vi "testtime.vi"() -> ()   [LabVIEW 2022 SP3]
panel:
  out "error out 8":errorcluster
  out "error out 7":errorcluster
  out "error out 6":errorcluster
  out "error out 5":errorcluster
  out "error out 4":errorcluster
  out "1 28":dbl format="%04d"
  out "1 27":dbl format="%04d"
  out "1 26":dbl format="%04d"
  out "1 25":dbl format="%04d"
  out "1 24":dbl format="%04d"
  out "1 23":dbl format="%04d"
  out "1 22":dbl format="%04d"
  out "error out 3":errorcluster
  out "1 21":dbl format="%04d"
  out "1 20":dbl format="%04d"
  out "1 19":dbl format="%04d"
  out "1 18":dbl format="%04d"
  out "1 17":dbl format="%04d"
  out "1 16":dbl format="%04d"
  out "1 15":dbl format="%04d"
  out "1 14":dbl format="%04d"
  out "1 13":dbl format="%04d"
  out "1 12":dbl format="%04d"
  out "1 11":dbl format="%04d"
  out "1 10":dbl format="%04d"
  out "1 9":dbl format="%04d"
  out "1 8":dbl format="%04d"
  out "error out 2":errorcluster
  in  "8":bool
  out "1 7":dbl format="%04d"
  out "1 6":dbl format="%04d"
  out "1 5":dbl format="%04d"
  out "1 4":dbl format="%04d"
  out "1 3":dbl format="%04d"
  out "1 2":dbl format="%04d"
  out "1":dbl format="%04d"
  out "error out":errorcluster
  # "A"
  # "B"
  # "C"
  # "D"
  # "11."
  # "Time"
  # "Setting"
  # "12."
  # "13."
  # "14."
  # "15."
  # "16."
  # "21."
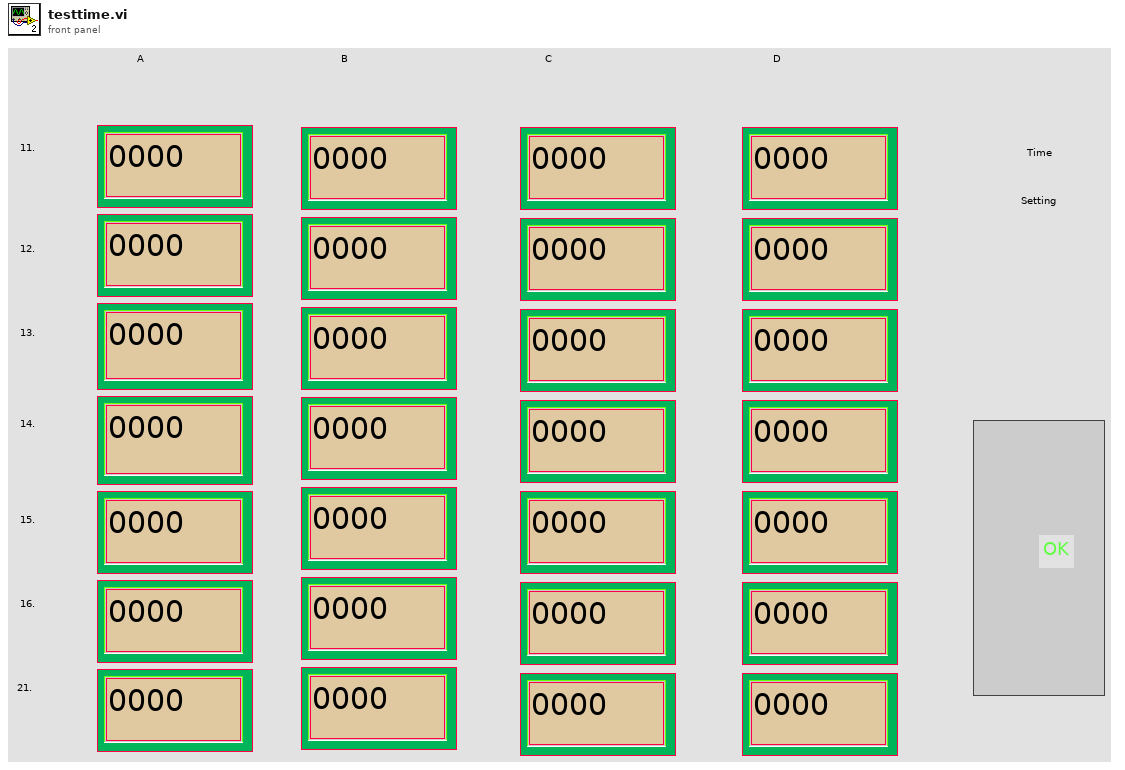
[diagram p1: front panel]
types:
  T1 = enum16{"open", "replace", "create", "open or create", "replace or create", "replace or create with confirmation"}
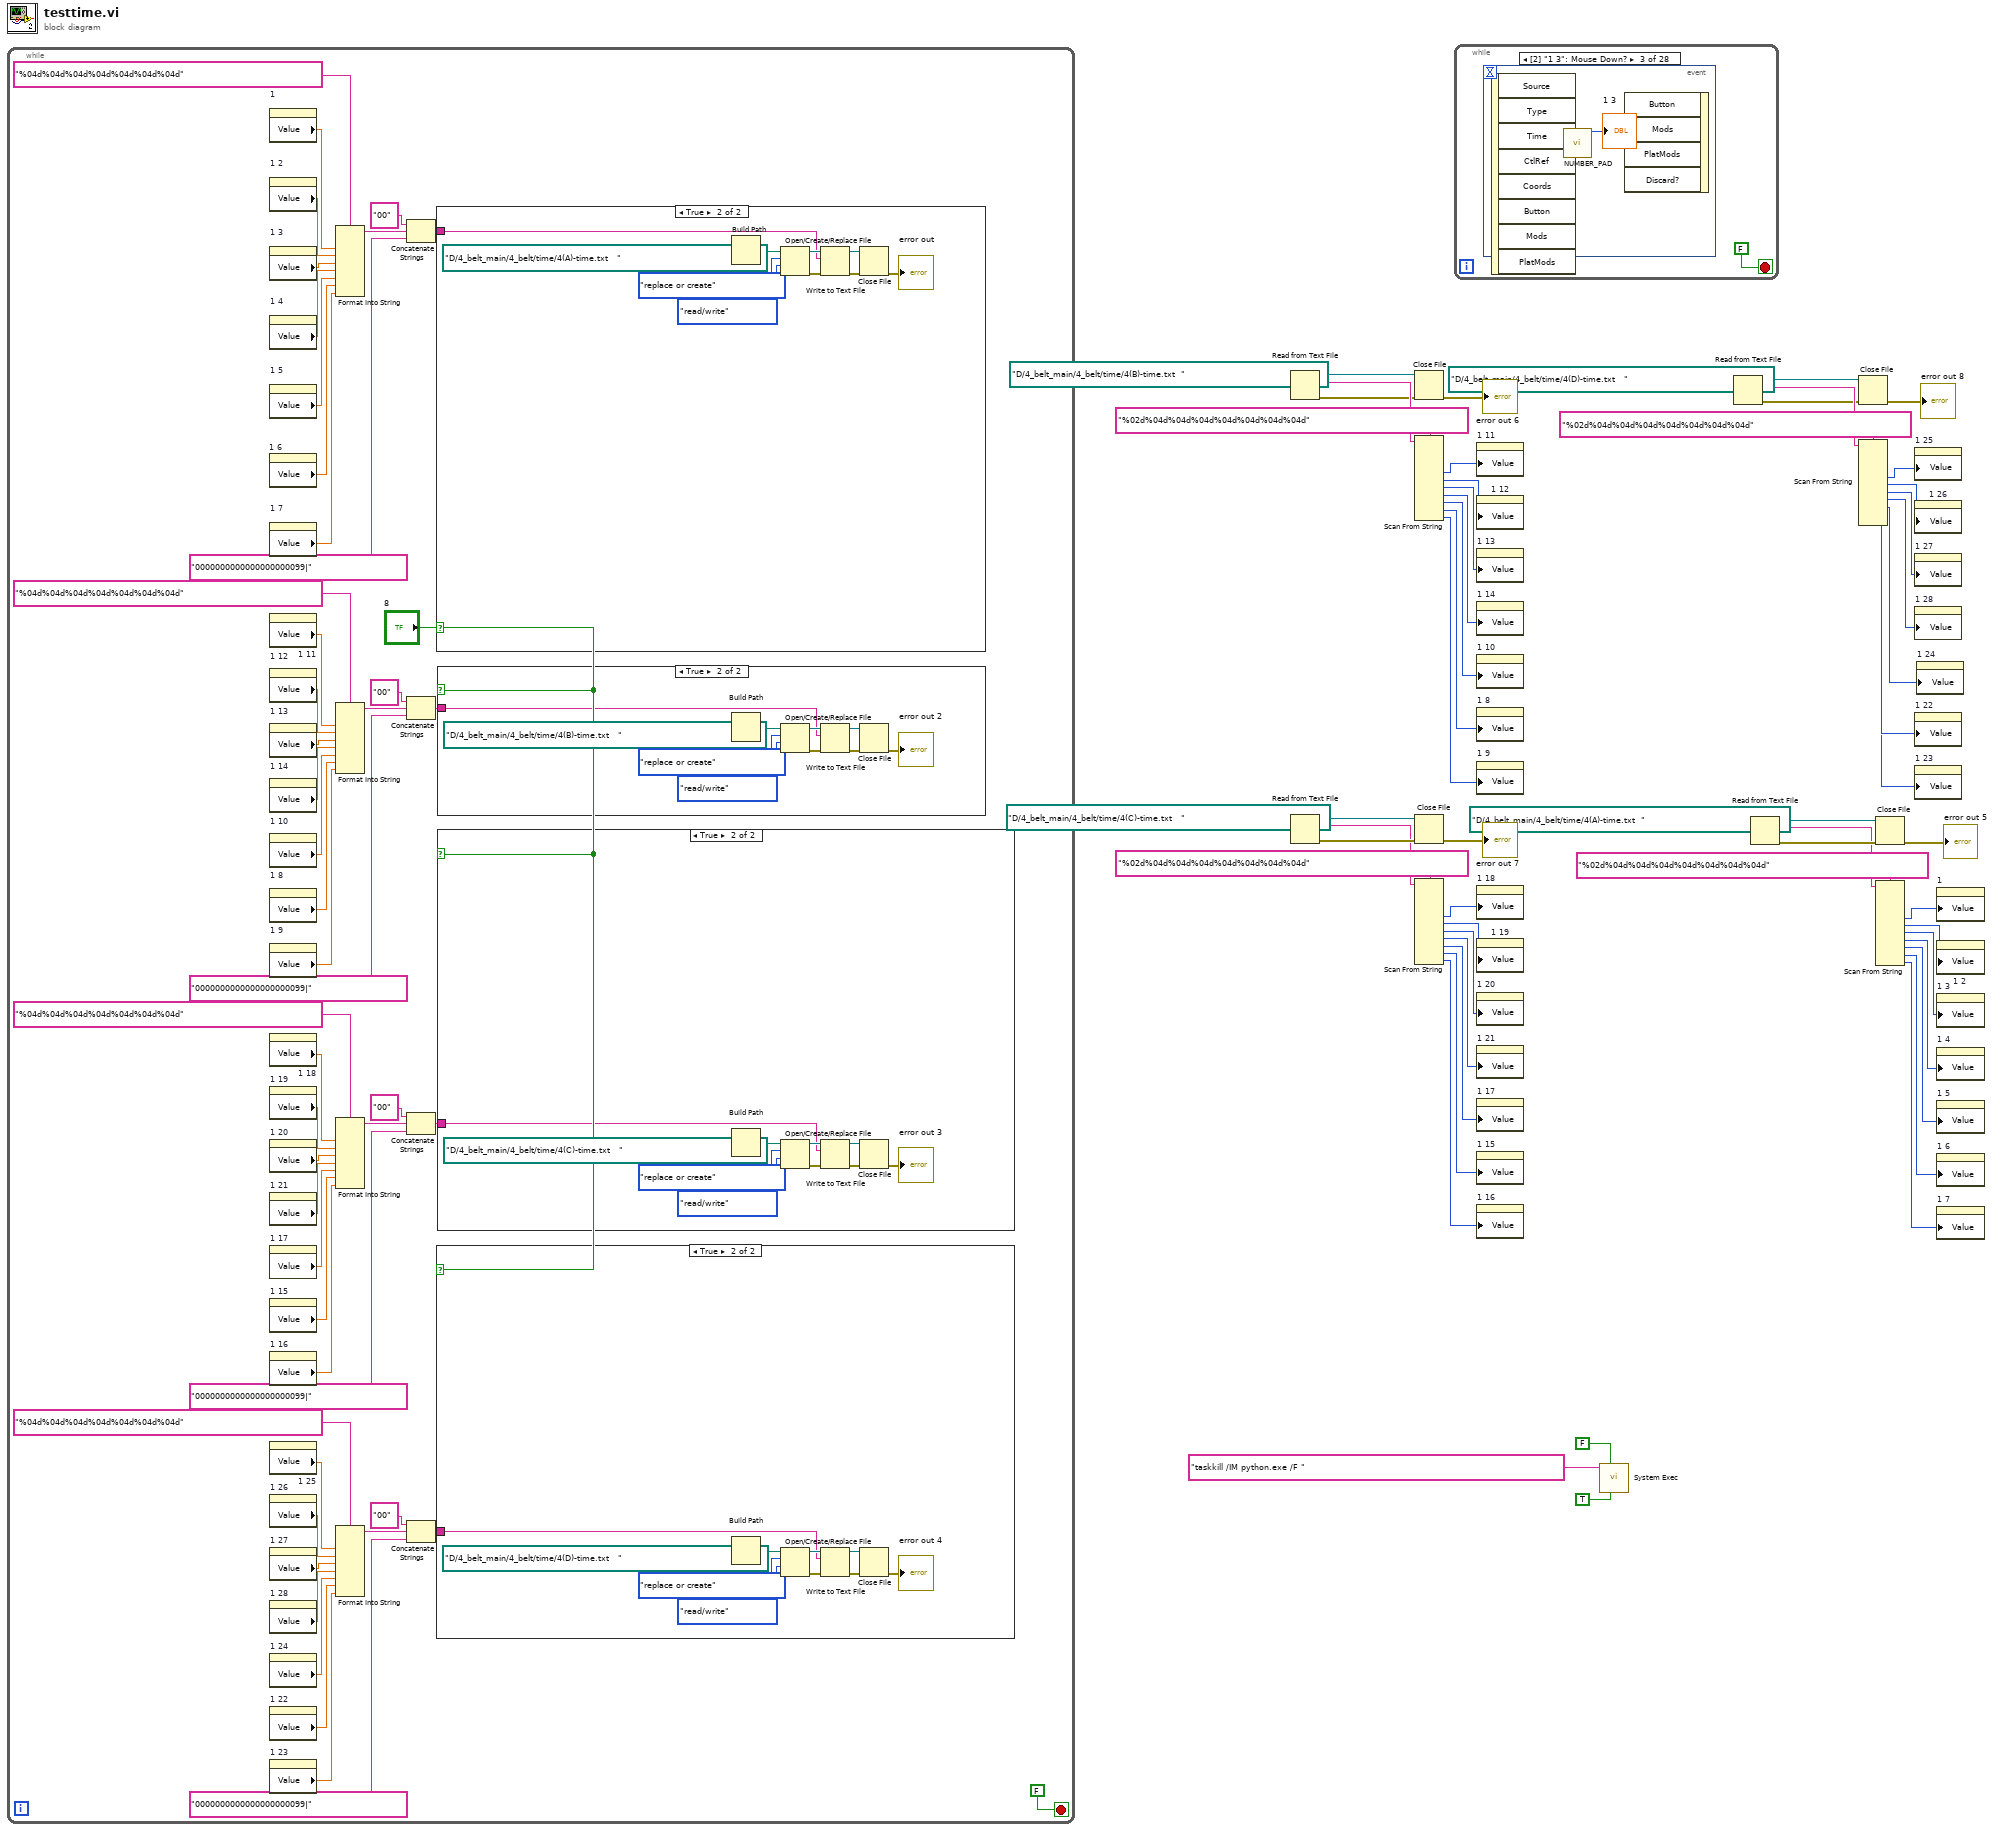
[diagram p0: block diagram]
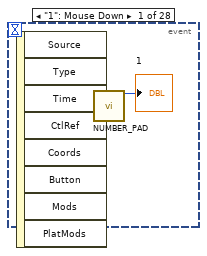
[diagram p2: hidden frame]
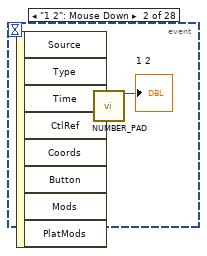
[diagram p3: hidden frame]
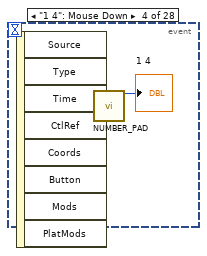
[diagram p4: hidden frame]
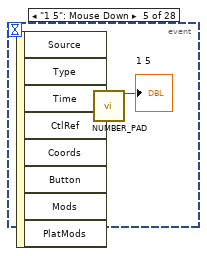
[diagram p5: hidden frame]
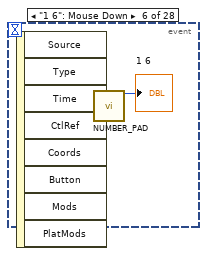
[diagram p6: hidden frame]
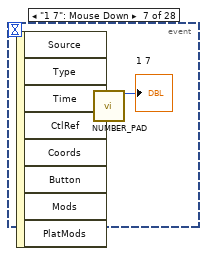
[diagram p7: hidden frame]
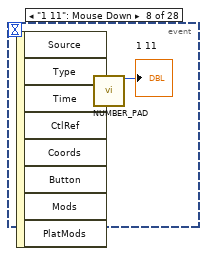
[diagram p8: hidden frame]
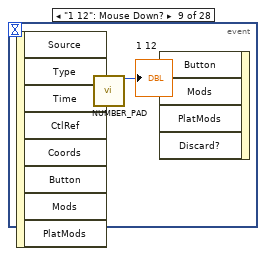
[diagram p9: hidden frame]
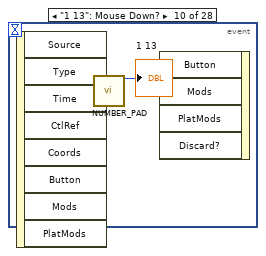
[diagram p10: hidden frame]
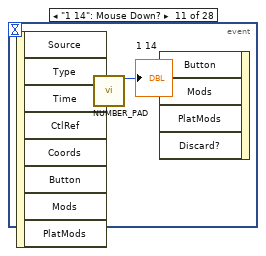
[diagram p11: hidden frame]
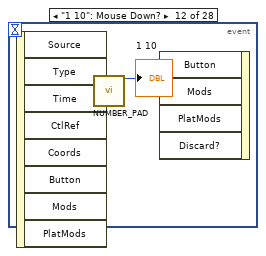
[diagram p12: hidden frame]
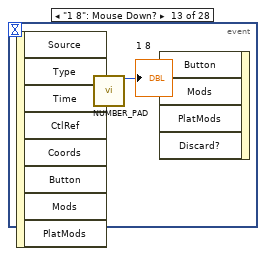
[diagram p13: hidden frame]
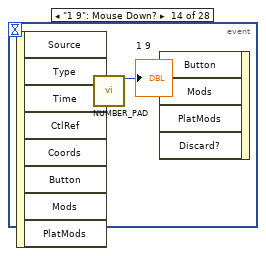
[diagram p14: hidden frame]
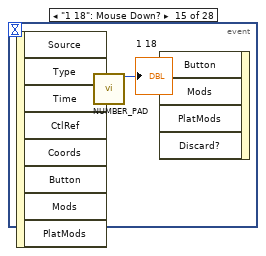
[diagram p15: hidden frame]
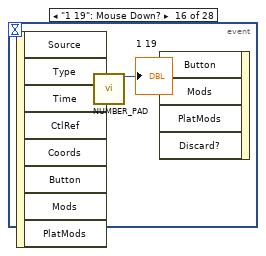
[diagram p16: hidden frame]
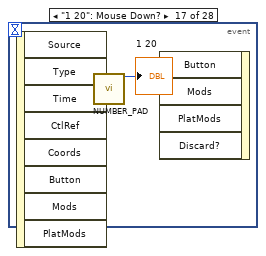
[diagram p17: hidden frame]
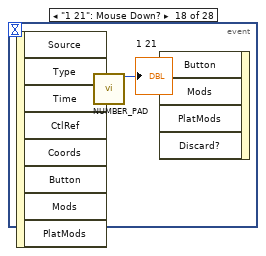
[diagram p18: hidden frame]
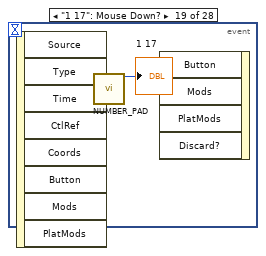
[diagram p19: hidden frame]
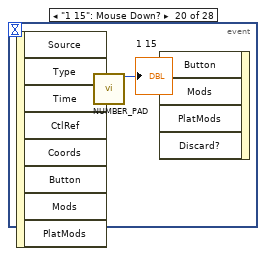
[diagram p20: hidden frame]
diagram:
  n1 = while {
    stop <- FALSE stop-if-true
    n2 = property on="1" class="DigNum (strict)"() -> ("Value"=w104:dbl)  [unwired: 2 in, 2 out]
    n3 = property on="1 2" class="DigNum (strict)"() -> ("Value"=w103:dbl)  [unwired: 2 in, 2 out]
    n4 = property on="1 3" class="DigNum (strict)"() -> ("Value"=w102:dbl)  [unwired: 2 in, 2 out]
    n5 = property on="1 4" class="DigNum (strict)"() -> ("Value"=w101:dbl)  [unwired: 2 in, 2 out]
    n6 = property on="1 5" class="DigNum (strict)"() -> ("Value"=w100:dbl)  [unwired: 2 in, 2 out]
    n7 = property on="1 6" class="DigNum (strict)"() -> ("Value"=w99:dbl)  [unwired: 2 in, 2 out]
    n8 = property on="1 7" class="DigNum (strict)"() -> ("Value"=w98:dbl)  [unwired: 2 in, 2 out]
    n9 = property on="1 11" class="DigNum (strict)"() -> ("Value"=w95:dbl)  [unwired: 2 in, 2 out]
    n10 = property on="1 12" class="DigNum (strict)"() -> ("Value"=w94:dbl)  [unwired: 2 in, 2 out]
    n11 = property on="1 13" class="DigNum (strict)"() -> ("Value"=w93:dbl)  [unwired: 2 in, 2 out]
    n12 = property on="1 14" class="DigNum (strict)"() -> ("Value"=w92:dbl)  [unwired: 2 in, 2 out]
    n13 = property on="1 10" class="DigNum (strict)"() -> ("Value"=w91:dbl)  [unwired: 2 in, 2 out]
    n14 = property on="1 8" class="DigNum (strict)"() -> ("Value"=w90:dbl)  [unwired: 2 in, 2 out]
    n15 = property on="1 9" class="DigNum (strict)"() -> ("Value"=w89:dbl)  [unwired: 2 in, 2 out]
    n16 = property on="1 18" class="DigNum (strict)"() -> ("Value"=w87:dbl)  [unwired: 2 in, 2 out]
    n17 = property on="1 19" class="DigNum (strict)"() -> ("Value"=w86:dbl)  [unwired: 2 in, 2 out]
    n18 = property on="1 20" class="DigNum (strict)"() -> ("Value"=w85:dbl)  [unwired: 2 in, 2 out]
    n19 = property on="1 21" class="DigNum (strict)"() -> ("Value"=w84:dbl)  [unwired: 2 in, 2 out]
    n20 = property on="1 17" class="DigNum (strict)"() -> ("Value"=w83:dbl)  [unwired: 2 in, 2 out]
    n21 = property on="1 15" class="DigNum (strict)"() -> ("Value"=w82:dbl)  [unwired: 2 in, 2 out]
    n22 = property on="1 16" class="DigNum (strict)"() -> ("Value"=w81:dbl)  [unwired: 2 in, 2 out]
    n23 = property on="1 25" class="DigNum (strict)"() -> ("Value"=w79:dbl)  [unwired: 2 in, 2 out]
    n24 = property on="1 26" class="DigNum (strict)"() -> ("Value"=w78:dbl)  [unwired: 2 in, 2 out]
    n25 = property on="1 27" class="DigNum (strict)"() -> ("Value"=w77:dbl)  [unwired: 2 in, 2 out]
    n26 = property on="1 28" class="DigNum (strict)"() -> ("Value"=w76:dbl)  [unwired: 2 in, 2 out]
    n27 = property on="1 24" class="DigNum (strict)"() -> ("Value"=w75:dbl)  [unwired: 2 in, 2 out]
    n28 = property on="1 22" class="DigNum (strict)"() -> ("Value"=w74:dbl)  [unwired: 2 in, 2 out]
    n29 = property on="1 23" class="DigNum (strict)"() -> ("Value"=w73:dbl)  [unwired: 2 in, 2 out]
    n30 = Format Into String(format string="%04d%04d%04d%04d%04d%04d%04d", w104, w103, w102, w101, w100, w99, w98) -> (resulting string=w72:string)  [unwired: 2 in, 1 out]
    n31 = Format Into String(format string="%04d%04d%04d%04d%04d%04d%04d", w95, w94, w93, w92, w91, w90, w89) -> (resulting string=w66:string)  [unwired: 2 in, 1 out]
    n32 = Format Into String(format string="%04d%04d%04d%04d%04d%04d%04d", w87, w86, w85, w84, w83, w82, w81) -> (resulting string=w62:string)  [unwired: 2 in, 1 out]
    n33 = Format Into String(format string="%04d%04d%04d%04d%04d%04d%04d", w79, w78, w77, w76, w75, w74, w73) -> (resulting string=w58:string)  [unwired: 2 in, 1 out]
    n34 = Concatenate Strings("00", w72, "0000000000000000000099|" ("string")) -> (w70:string)
    n35 = Concatenate Strings("00", w66, "0000000000000000000099|" ("string")) -> (w65:string)
    n36 = Concatenate Strings("00", w62, "0000000000000000000099|" ("string")) -> (w61:string)
    n37 = Concatenate Strings("00", w58, "0000000000000000000099|" ("string")) -> (w57:string)
    n38 = case shown="True" "8" {
      tunnel: w70 -> [_ w137]
      frame False {
      }
      frame True {
        n39 = Build Path(name or relative path=path "D:/4_belt_main/4_belt/time/4(A)-time.txt   ") -> (appended path=w145:path)  [unwired: 1 in]
        n40 = Open/Create/Replace File(file path (use dialog)=w145, operation (0:open)=T1."replace or create", access (0:read/write)=enum16{"read/write", "read-only", "write-only"}."read/write") -> (refnum out=w142:refnum<file>, error out=w141:errorcluster)  [unwired: 3 in, 1 out]
        n41 = Write to Text File(file (use dialog)=w142, text=w137, error in=w141) -> (refnum out=w140:refnum<file>, error out=w139:errorcluster)  [unwired: 1 in, 1 out]
        n42 = Close File(refnum=w140, error in=w139) -> (error out=→"error out":errorcluster)  [unwired: 1 out]
      }
    }
    n43 = case shown="True" "8" {
      tunnel: w57 -> [_ w106]
      frame False {
      }
      frame True {
        n44 = Build Path(name or relative path=path "D:/4_belt_main/4_belt/time/4(D)-time.txt   ") -> (appended path=w115:path)  [unwired: 1 in]
        n45 = Open/Create/Replace File(file path (use dialog)=w115, operation (0:open)=T1."replace or create", access (0:read/write)=enum16{"read/write", "read-only", "write-only"}."read/write") -> (refnum out=w112:refnum<file>, error out=w111:errorcluster)  [unwired: 3 in, 1 out]
        n46 = Write to Text File(file (use dialog)=w112, text=w106, error in=w111) -> (refnum out=w110:refnum<file>, error out=w109:errorcluster)  [unwired: 1 in, 1 out]
        n47 = Close File(refnum=w110, error in=w109) -> (error out=→"error out 4":errorcluster)  [unwired: 1 out]
      }
    }
    n48 = case shown="True" "8" {
      tunnel: w65 -> [_ w126]
      frame False {
      }
      frame True {
        n49 = Build Path(name or relative path=path "D:/4_belt_main/4_belt/time/4(B)-time.txt   ") -> (appended path=w135:path)  [unwired: 1 in]
        n50 = Open/Create/Replace File(file path (use dialog)=w135, operation (0:open)=T1."replace or create", access (0:read/write)=enum16{"read/write", "read-only", "write-only"}."read/write") -> (refnum out=w132:refnum<file>, error out=w131:errorcluster)  [unwired: 3 in, 1 out]
        n51 = Write to Text File(file (use dialog)=w132, text=w126, error in=w131) -> (refnum out=w130:refnum<file>, error out=w129:errorcluster)  [unwired: 1 in, 1 out]
        n52 = Close File(refnum=w130, error in=w129) -> (error out=→"error out 2":errorcluster)  [unwired: 1 out]
      }
    }
    n53 = case shown="True" "8" {
      tunnel: w61 -> [_ w116]
      frame False {
      }
      frame True {
        n54 = Build Path(name or relative path=path "D:/4_belt_main/4_belt/time/4(C)-time.txt   ") -> (appended path=w125:path)  [unwired: 1 in]
        n55 = Open/Create/Replace File(file path (use dialog)=w125, operation (0:open)=T1."replace or create", access (0:read/write)=enum16{"read/write", "read-only", "write-only"}."read/write") -> (refnum out=w122:refnum<file>, error out=w121:errorcluster)  [unwired: 3 in, 1 out]
        n56 = Write to Text File(file (use dialog)=w122, text=w116, error in=w121) -> (refnum out=w120:refnum<file>, error out=w119:errorcluster)  [unwired: 1 in, 1 out]
        n57 = Close File(refnum=w120, error in=w119) -> (error out=→"error out 3":errorcluster)  [unwired: 1 out]
      }
    }
  }
  n58 = Read from Text File(file (use dialog)=path "D:/4_belt_main/4_belt/time/4(B)-time.txt  " ("name or relative path")) -> (refnum out=w37:refnum<file>, text=w41:string, error out=w38:errorcluster)  [unwired: 3 in, 1 out]
  n59 = Read from Text File(file (use dialog)=path "D:/4_belt_main/4_belt/time/4(C)-time.txt   " ("name or relative path")) -> (refnum out=w29:refnum<file>, text=w25:string, error out=w28:errorcluster)  [unwired: 3 in, 1 out]
  n60 = Close File(refnum=w37, error in=w38) -> (error out=→"error out 6":errorcluster)  [unwired: 1 out]
  n61 = Scan From String(format string="%02d%04d%04d%04d%04d%04d%04d%04d", input string=w41) -> (output 2=w36:i32, output 3=w35:i32, output 4=w34:i32, output 5=w33:i32, output 6=w32:i32, output 7=w31:i32, output 8=w30:i32)  [unwired: 11 in, 3 out]
  n62 = Close File(refnum=w29, error in=w28) -> (error out=→"error out 7":errorcluster)  [unwired: 1 out]
  n63 = Scan From String(format string="%02d%04d%04d%04d%04d%04d%04d%04d", input string=w25) -> (output 2=w23:i32, output 3=w22:i32, output 4=w21:i32, output 5=w20:i32, output 6=w19:i32, output 7=w18:i32, output 8=w17:i32)  [unwired: 11 in, 3 out]
  n64 = while {
    stop <- FALSE stop-if-true
    n65 = event shown="[2] \"1 3\": Mouse Down?" {
      selector: _ -> [_ _ _ _ _ _ _ _ _ _ _ _ _ _ _ _ _ _ _ _ _ _ _ _ _ _ _ _]
      dyn-events: _ -> [_ _ _ _ _ _ _ _ _ _ _ _ _ _ _ _ _ _ _ _ _ _ _ _ _ _ _ _]
      timeout: _ -> [_ _ _ _ _ _ _ _ _ _ _ _ _ _ _ _ _ _ _ _ _ _ _ _ _ _ _ _]
      event "1": Mouse Down {
        n66 = event-data() -> ()  [unwired: 1 in, 8 out]
        n67 = call "NUMBER_PAD.vi"() -> ("number (out)"=→"1":i32)  [unwired: 15 in]
      }
      event "1 2": Mouse Down {
        n68 = event-data() -> ()  [unwired: 1 in, 8 out]
        n69 = call "NUMBER_PAD.vi"() -> ("number (out)"=→"1 2":i32)  [unwired: 15 in]
      }
      event "1 3": Mouse Down? {
        n70 = event-data() -> ()  [unwired: 1 in, 8 out]
        n71 = call "NUMBER_PAD.vi"() -> ("number (out)"=→"1 3":i32)  [unwired: 15 in]
        n72 = event-data() -> ()  [unwired: 5 in, 1 out]
      }
      event "1 4": Mouse Down {
        n73 = event-data() -> ()  [unwired: 1 in, 8 out]
        n74 = call "NUMBER_PAD.vi"() -> ("number (out)"=→"1 4":i32)  [unwired: 15 in]
      }
      event "1 5": Mouse Down {
        n75 = event-data() -> ()  [unwired: 1 in, 8 out]
        n76 = call "NUMBER_PAD.vi"() -> ("number (out)"=→"1 5":i32)  [unwired: 15 in]
      }
      event "1 6": Mouse Down {
        n77 = event-data() -> ()  [unwired: 1 in, 8 out]
        n78 = call "NUMBER_PAD.vi"() -> ("number (out)"=→"1 6":i32)  [unwired: 15 in]
      }
      event "1 7": Mouse Down {
        n79 = event-data() -> ()  [unwired: 1 in, 8 out]
        n80 = call "NUMBER_PAD.vi"() -> ("number (out)"=→"1 7":i32)  [unwired: 15 in]
      }
      event "1 11": Mouse Down {
        n81 = event-data() -> ()  [unwired: 1 in, 8 out]
        n82 = call "NUMBER_PAD.vi"() -> ("number (out)"=→"1 11":i32)  [unwired: 15 in]
      }
      event "1 12": Mouse Down? {
        n83 = event-data() -> ()  [unwired: 1 in, 8 out]
        n84 = call "NUMBER_PAD.vi"() -> ("number (out)"=→"1 12":i32)  [unwired: 15 in]
        n85 = event-data() -> ()  [unwired: 5 in, 1 out]
      }
      event "1 13": Mouse Down? {
        n86 = event-data() -> ()  [unwired: 1 in, 8 out]
        n87 = call "NUMBER_PAD.vi"() -> ("number (out)"=→"1 13":i32)  [unwired: 15 in]
        n88 = event-data() -> ()  [unwired: 5 in, 1 out]
      }
      event "1 14": Mouse Down? {
        n89 = event-data() -> ()  [unwired: 1 in, 8 out]
        n90 = call "NUMBER_PAD.vi"() -> ("number (out)"=→"1 14":i32)  [unwired: 15 in]
        n91 = event-data() -> ()  [unwired: 5 in, 1 out]
      }
      event "1 10": Mouse Down? {
        n92 = event-data() -> ()  [unwired: 1 in, 8 out]
        n93 = call "NUMBER_PAD.vi"() -> ("number (out)"=→"1 10":i32)  [unwired: 15 in]
        n94 = event-data() -> ()  [unwired: 5 in, 1 out]
      }
      event "1 8": Mouse Down? {
        n95 = event-data() -> ()  [unwired: 1 in, 8 out]
        n96 = call "NUMBER_PAD.vi"() -> ("number (out)"=→"1 8":i32)  [unwired: 15 in]
        n97 = event-data() -> ()  [unwired: 5 in, 1 out]
      }
      event "1 9": Mouse Down? {
        n98 = event-data() -> ()  [unwired: 1 in, 8 out]
        n99 = call "NUMBER_PAD.vi"() -> ("number (out)"=→"1 9":i32)  [unwired: 15 in]
        n100 = event-data() -> ()  [unwired: 5 in, 1 out]
      }
      event "1 18": Mouse Down? {
        n101 = event-data() -> ()  [unwired: 1 in, 8 out]
        n102 = call "NUMBER_PAD.vi"() -> ("number (out)"=→"1 18":i32)  [unwired: 15 in]
        n103 = event-data() -> ()  [unwired: 5 in, 1 out]
      }
      event "1 19": Mouse Down? {
        n104 = event-data() -> ()  [unwired: 1 in, 8 out]
        n105 = call "NUMBER_PAD.vi"() -> ("number (out)"=→"1 19":i32)  [unwired: 15 in]
        n106 = event-data() -> ()  [unwired: 5 in, 1 out]
      }
      event "1 20": Mouse Down? {
        n107 = event-data() -> ()  [unwired: 1 in, 8 out]
        n108 = call "NUMBER_PAD.vi"() -> ("number (out)"=→"1 20":i32)  [unwired: 15 in]
        n109 = event-data() -> ()  [unwired: 5 in, 1 out]
      }
      event "1 21": Mouse Down? {
        n110 = event-data() -> ()  [unwired: 1 in, 8 out]
        n111 = call "NUMBER_PAD.vi"() -> ("number (out)"=→"1 21":i32)  [unwired: 15 in]
        n112 = event-data() -> ()  [unwired: 5 in, 1 out]
      }
      event "1 17": Mouse Down? {
        n113 = event-data() -> ()  [unwired: 1 in, 8 out]
        n114 = call "NUMBER_PAD.vi"() -> ("number (out)"=→"1 17":i32)  [unwired: 15 in]
        n115 = event-data() -> ()  [unwired: 5 in, 1 out]
      }
      event "1 15": Mouse Down? {
        n116 = event-data() -> ()  [unwired: 1 in, 8 out]
        n117 = call "NUMBER_PAD.vi"() -> ("number (out)"=→"1 15":i32)  [unwired: 15 in]
        n118 = event-data() -> ()  [unwired: 5 in, 1 out]
      }
      event "1 16": Mouse Down? {
        n119 = event-data() -> ()  [unwired: 1 in, 8 out]
        n120 = call "NUMBER_PAD.vi"() -> ("number (out)"=→"1 16":i32)  [unwired: 15 in]
        n121 = event-data() -> ()  [unwired: 5 in, 1 out]
      }
      event "1 25": Mouse Down? {
        n122 = event-data() -> ()  [unwired: 1 in, 8 out]
        n123 = call "NUMBER_PAD.vi"() -> ("number (out)"=→"1 25":i32)  [unwired: 15 in]
        n124 = event-data() -> ()  [unwired: 5 in, 1 out]
      }
      event "1 26": Mouse Down? {
        n125 = event-data() -> ()  [unwired: 1 in, 8 out]
        n126 = call "NUMBER_PAD.vi"() -> ("number (out)"=→"1 26":i32)  [unwired: 15 in]
        n127 = event-data() -> ()  [unwired: 5 in, 1 out]
      }
      event "1 27": Mouse Down? {
        n128 = event-data() -> ()  [unwired: 1 in, 8 out]
        n129 = call "NUMBER_PAD.vi"() -> ("number (out)"=→"1 27":i32)  [unwired: 15 in]
        n130 = event-data() -> ()  [unwired: 5 in, 1 out]
      }
      event "1 28": Mouse Down? {
        n131 = event-data() -> ()  [unwired: 1 in, 8 out]
        n132 = call "NUMBER_PAD.vi"() -> ("number (out)"=→"1 28":i32)  [unwired: 15 in]
        n133 = event-data() -> ()  [unwired: 5 in, 1 out]
      }
      event "1 24": Mouse Down? {
        n134 = event-data() -> ()  [unwired: 1 in, 8 out]
        n135 = call "NUMBER_PAD.vi"() -> ("number (out)"=→"1 24":i32)  [unwired: 15 in]
        n136 = event-data() -> ()  [unwired: 5 in, 1 out]
      }
      event "1 22": Mouse Down? {
        n137 = event-data() -> ()  [unwired: 1 in, 8 out]
        n138 = call "NUMBER_PAD.vi"() -> ("number (out)"=→"1 22":i32)  [unwired: 15 in]
        n139 = event-data() -> ()  [unwired: 5 in, 1 out]
      }
      event "1 23": Mouse Down? {
        n140 = event-data() -> ()  [unwired: 1 in, 8 out]
        n141 = call "NUMBER_PAD.vi"() -> ("number (out)"=→"1 23":i32)  [unwired: 15 in]
        n142 = event-data() -> ()  [unwired: 5 in, 1 out]
      }
    }
  }
  n143 = property on="1 11" class="DigNum (strict)"("Value"=w36) -> ()  [unwired: 2 in, 2 out]
  n144 = property on="1 12" class="DigNum (strict)"("Value"=w35) -> ()  [unwired: 2 in, 2 out]
  n145 = property on="1 13" class="DigNum (strict)"("Value"=w34) -> ()  [unwired: 2 in, 2 out]
  n146 = property on="1 14" class="DigNum (strict)"("Value"=w33) -> ()  [unwired: 2 in, 2 out]
  n147 = property on="1 10" class="DigNum (strict)"("Value"=w32) -> ()  [unwired: 2 in, 2 out]
  n148 = property on="1 8" class="DigNum (strict)"("Value"=w31) -> ()  [unwired: 2 in, 2 out]
  n149 = property on="1 9" class="DigNum (strict)"("Value"=w30) -> ()  [unwired: 2 in, 2 out]
  n150 = property on="1 18" class="DigNum (strict)"("Value"=w23) -> ()  [unwired: 2 in, 2 out]
  n151 = property on="1 19" class="DigNum (strict)"("Value"=w22) -> ()  [unwired: 2 in, 2 out]
  n152 = property on="1 20" class="DigNum (strict)"("Value"=w21) -> ()  [unwired: 2 in, 2 out]
  n153 = property on="1 21" class="DigNum (strict)"("Value"=w20) -> ()  [unwired: 2 in, 2 out]
  n154 = property on="1 17" class="DigNum (strict)"("Value"=w19) -> ()  [unwired: 2 in, 2 out]
  n155 = property on="1 15" class="DigNum (strict)"("Value"=w18) -> ()  [unwired: 2 in, 2 out]
  n156 = property on="1 16" class="DigNum (strict)"("Value"=w17) -> ()  [unwired: 2 in, 2 out]
  n157 = call <vilib>:"System Exec.vi"("run minimized? (F)"=TRUE, "wait until completion? (T)"=FALSE, "command line"="taskkill /IM python.exe /F ") -> ()  [unwired: 5 in, 4 out]
  n158 = Read from Text File(file (use dialog)=path "D:/4_belt_main/4_belt/time/4(D)-time.txt   " ("name or relative path")) -> (refnum out=w11:refnum<file>, text=w15:string, error out=w12:errorcluster)  [unwired: 3 in, 1 out]
  n159 = Read from Text File(file (use dialog)=path "D:/4_belt_main/4_belt/time/4(A)-time.txt  " ("name or relative path")) -> (refnum out=w55:refnum<file>, text=w51:string, error out=w54:errorcluster)  [unwired: 3 in, 1 out]
  n160 = Close File(refnum=w11, error in=w12) -> (error out=→"error out 8":errorcluster)  [unwired: 1 out]
  n161 = Scan From String(format string="%02d%04d%04d%04d%04d%04d%04d%04d", input string=w15) -> (output 2=w10:i32, output 3=w9:i32, output 4=w8:i32, output 5=w7:i32, output 6=w6:i32, output 7=w5:i32, output 8=w4:i32)  [unwired: 11 in, 3 out]
  n162 = Close File(refnum=w55, error in=w54) -> (error out=→"error out 5":errorcluster)  [unwired: 1 out]
  n163 = Scan From String(format string="%02d%04d%04d%04d%04d%04d%04d%04d", input string=w51) -> (output 2=w49:i32, output 3=w48:i32, output 4=w47:i32, output 5=w46:i32, output 6=w45:i32, output 7=w44:i32, output 8=w43:i32)  [unwired: 11 in, 3 out]
  n164 = property on="1 25" class="DigNum (strict)"("Value"=w10) -> ()  [unwired: 2 in, 2 out]
  n165 = property on="1 26" class="DigNum (strict)"("Value"=w9) -> ()  [unwired: 2 in, 2 out]
  n166 = property on="1 27" class="DigNum (strict)"("Value"=w8) -> ()  [unwired: 2 in, 2 out]
  n167 = property on="1 28" class="DigNum (strict)"("Value"=w7) -> ()  [unwired: 2 in, 2 out]
  n168 = property on="1 22" class="DigNum (strict)"("Value"=w5) -> ()  [unwired: 2 in, 2 out]
  n169 = property on="1 23" class="DigNum (strict)"("Value"=w4) -> ()  [unwired: 2 in, 2 out]
  n170 = property on="1 24" class="DigNum (strict)"("Value"=w6) -> ()  [unwired: 2 in, 2 out]
  n171 = property on="1" class="DigNum (strict)"("Value"=w49) -> ()  [unwired: 2 in, 2 out]
  n172 = property on="1 2" class="DigNum (strict)"("Value"=w48) -> ()  [unwired: 2 in, 2 out]
  n173 = property on="1 3" class="DigNum (strict)"("Value"=w47) -> ()  [unwired: 2 in, 2 out]
  n174 = property on="1 4" class="DigNum (strict)"("Value"=w46) -> ()  [unwired: 2 in, 2 out]
  n175 = property on="1 5" class="DigNum (strict)"("Value"=w45) -> ()  [unwired: 2 in, 2 out]
  n176 = property on="1 6" class="DigNum (strict)"("Value"=w44) -> ()  [unwired: 2 in, 2 out]
  n177 = property on="1 7" class="DigNum (strict)"("Value"=w43) -> ()  [unwired: 2 in, 2 out]
